vi "select suggested protocols.vi"(10 "Codes":T2) -> (2 "To blink PN's":T1)   [LabVIEW 2011]
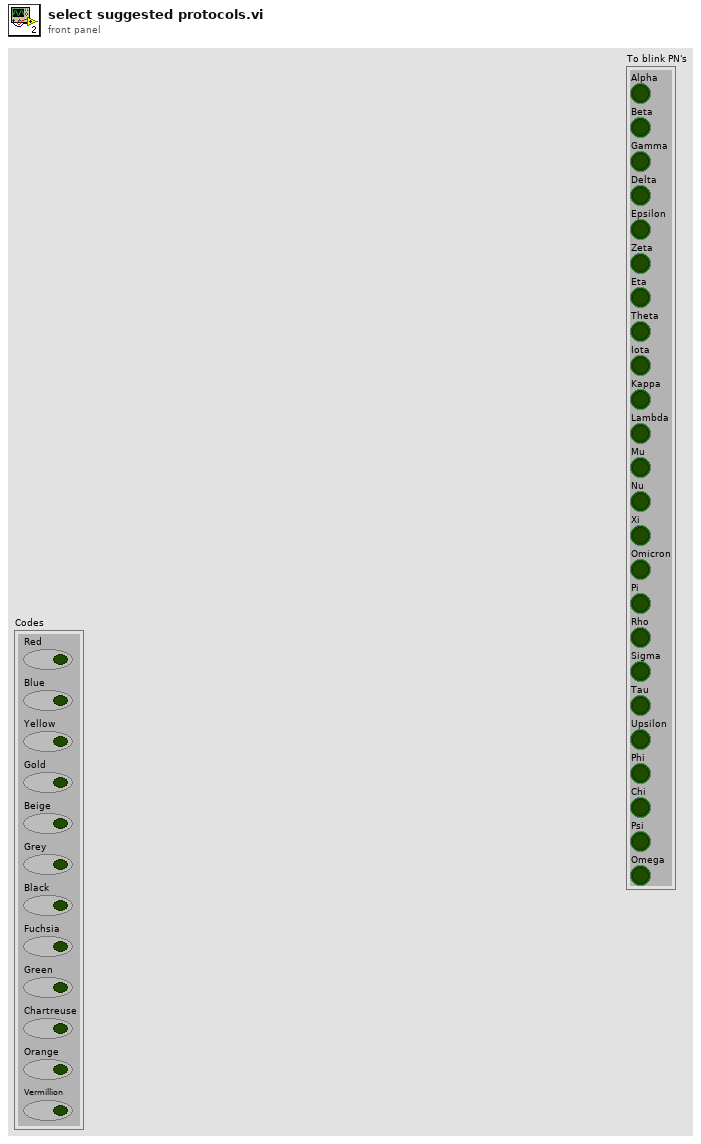
[diagram p1: front panel]
types:
  T1 = cluster{"Alpha":bool, "Beta":bool, "Gamma":bool, "Delta":bool, "Epsilon":bool, "Zeta":bool, "Eta":bool, "Theta":bool, "Iota":bool, "Kappa":bool, "Lambda":bool, "Mu":bool, "Nu":bool, "Xi":bool, "Omicron":bool, "Pi":bool, "Rho":bool, "Sigma":bool, "Tau":bool, "Upsilon":bool, "Phi":bool, "Chi":bool, "Psi":bool, "Omega":bool}
  T2 = cluster{"Red":bool, "Blue":bool, "Yellow":bool, "Gold":bool, "Beige":bool, "Grey":bool, "Black":bool, "Fuchsia":bool, "Green":bool, "Chartreuse":bool, "Orange":bool, "Vermillion":bool}
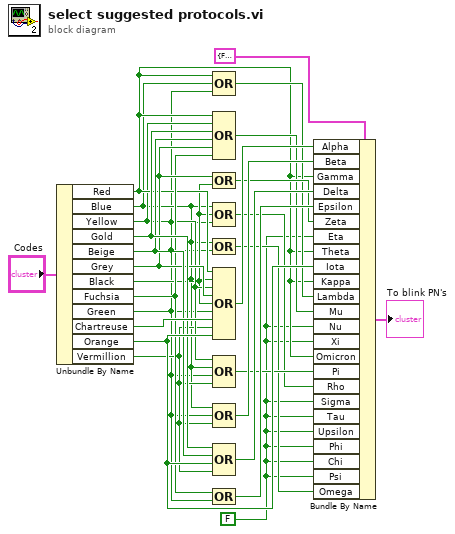
[diagram p0: block diagram]
diagram:
  w1 = FALSE
  n1 = Unbundle By Name("Codes") -> ("Red"=w11:bool, "Blue"=w4:bool, "Yellow"=w9:bool, "Gold"=w15:bool, "Beige"=w14:bool, "Grey"=w13:bool, "Black"=w6:bool, "Fuchsia"=w12:bool, "Green"=w3:bool, "Chartreuse"=w23:bool, "Orange"=w18:bool, "Vermillion"=w8:bool)
  n2 = Compound Arithmetic op=OR(w11, w4, w3) -> (w17:bool)
  n3 = Compound Arithmetic op=OR(w11, w9, w15, w14, w13, w12) -> (w16:bool)
  n4 = Compound Arithmetic op=OR(w13, w6) -> (w19:bool)
  n5 = Compound Arithmetic op=OR(w4, w6, w3) -> (w7:bool)
  n6 = Compound Arithmetic op=OR(w4, w3) -> (w5:bool)
  n7 = Compound Arithmetic op=OR(w11, w4, w9, w13, w6, w3, w23, w8, w18) -> (w24:bool)
  n8 = Compound Arithmetic op=OR(w9, w4, w3, w8) -> (w10:bool)
  n9 = Compound Arithmetic op=OR(w4, w3, w8) -> (w22:bool)
  n10 = Compound Arithmetic op=OR(w15, w14, w18, w8) -> (w21:bool)
  n11 = Compound Arithmetic op=OR(w12, w3) -> (w20:bool)
  n12 = Bundle By Name(cluster=T1 {"Alpha"=FALSE, "Beta"=FALSE, "Gamma"=FALSE, "Delta"=FALSE, "Epsilon"=FALSE, "Zeta"=FALSE, "Eta"=FALSE, "Theta"=FALSE, "Iota"=FALSE, "Kappa"=FALSE, "Lambda"=FALSE, "Mu"=FALSE, "Nu"=FALSE, "Xi"=FALSE, "Omicron"=FALSE, "Pi"=FALSE, "Rho"=FALSE, "Sigma"=FALSE, "Tau"=FALSE, "Upsilon"=FALSE, "Phi"=FALSE, "Chi"=FALSE, "Psi"=FALSE, "Omega"=FALSE}, "Alpha"=w24, "Beta"=w22, "Gamma"=w11, "Delta"=w21, "Epsilon"=w20, "Zeta"=w19, "Eta"=w1, "Theta"=w11, "Iota"=w18, "Kappa"=w11, "Lambda"=w17, "Mu"=w16, "Nu"=w1, "Xi"=w1, "Omicron"=w11, "Pi"=w10, "Rho"=w7, "Sigma"=w1, "Tau"=w1, "Upsilon"=w1, "Phi"=w1, "Chi"=w1, "Psi"=w1, "Omega"=w5) -> (→"To blink PN's":T1)
